vi "CheckWorkingRange.vi"(7 "channel status in":string, 8 "error in (no error)":errorcluster, 9 "Working Current":T2, 11 "Map in":T1) -> (0 "error out":errorcluster, 2 "in range?":bool, 3 "Map out":T1, 5 "channel status out":string)   [LabVIEW 2017, in "McsaAnalysisLowRate.lvlib"]
uses:
  <vilib>/addons/InsightCM/Devices/Shared/Mcsa/McsaAnalysisLowRate/McsaAnalysisLowRate.lvlib
  <vilib>/addons/InsightCM/Utilities/Analysis/MCSA/controls/WorkingCurrent.ctl
  <vilib>/addons/PointValueMap/controls/PointMap.ctl
  <vilib>/addons/PointValueMap/PointValueMap.lvlib
  <vilib>/addons/InsightCM/Utilities/Analysis/MCSA/McsaAnalysisFunctions.lvlib
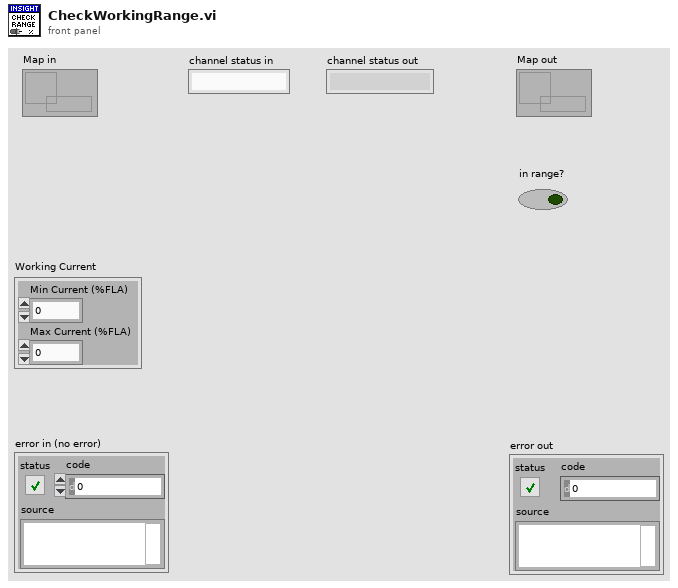
[diagram p1: front panel]
types:
  T1 = typedef "PointValueMap.lvlib/PointMap.ctl" = refnum<data-value>
  T2 = typedef "McsaAnalysisFunctions.lvlib/WorkingCurrent.ctl" = cluster{"Min Current (%FLA)":dbl, "Max Current (%FLA)":dbl}
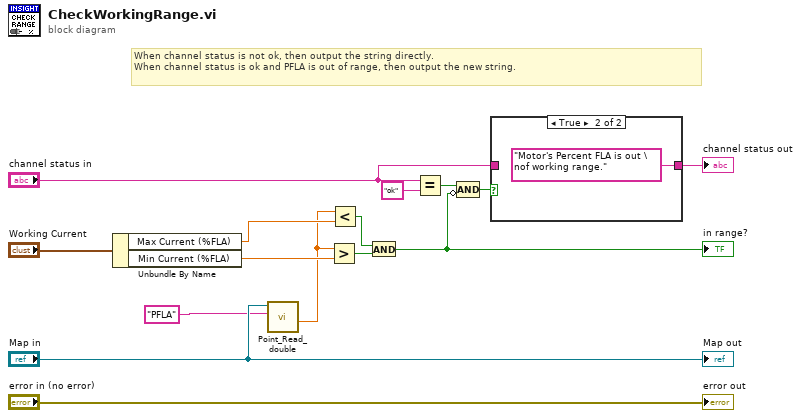
[diagram p0: block diagram]
diagram:
  # "When channel status is not ok, then output the string directly.\nWhen channel status is ok and PFLA is out of range, then output the new string."
  n1 = Unbundle By Name("Working Current") -> ("Max Current (%FLA)"=w11:dbl, "Min Current (%FLA)"=w12:dbl)
  n2 = call <vilib>:"Point_Read_double.vi"("Tag"="PFLA", "Map"="Map in") -> ("Value"=w10:dbl)  [unwired: 4 in, 5 out]
  n3 = Greater?(x=w10, y=w12) -> (0:w8:bool)
  n4 = Less?(x=w10, y=w11) -> (x < y?=w9:bool)
  n5 = And(x=w9, y=w8) -> (x .and. y?=w2:bool)
  "in range?" <- w2
  n6 = Equal?(x="channel status in", y="ok") -> (x = y?=w4:bool)
  n7 = Compound Arithmetic op=AND(w4, invert w2) -> (w5:bool)
  n8 = case shown="True" w5 {
    tunnel: [w16 "Motor's Percent FLA is out \nof working range."] -> w7
    tunnel: "channel status in" -> [w16 _]
    frame False {
    }
    frame True {
    }
  }
  "channel status out" <- w7
  "error out" <- "error in (no error)"
  "Map out" <- "Map in"
